vi "provide_OME_data.vi"(6 "image ID":string, 8 "error in (no error)":errorcluster, 9 "structuredAttribute string in":string, 10 "OME element in":refnum<class "XMLElement.lvclass">, 11 "InstrumentDL090324 in":refnum<class "InstrumentDL090324.lvclass">) -> (0 "error out":errorcluster, 1 "structuredAttribute string out":string, 2 "OME element out":refnum<class "XMLElement.lvclass">, 3 "InstrumentDL090324 out":refnum<class "InstrumentDL090324.lvclass">)   [LabVIEW 2010, in "InstrumentDL090324.lvclass"]
uses:
  InstrumentDL090324.lvclass
  common/classes/XMLElement/XMLElement/XMLElement.lvclass
  GenericInstrument/GenericInstrument/GenericInstrument.lvclass
  InstrumentDL090324.lvclass/InstrumentDL090324.ctl
  Detector/GenericDetector/GenericDetector/GenericDetector.lvclass
  LightSource/GenericLightSource/GenericLightSource/GenericLightSource.lvclass
  Objective/GenericObjective/GenericObjective/GenericObjective.lvclass
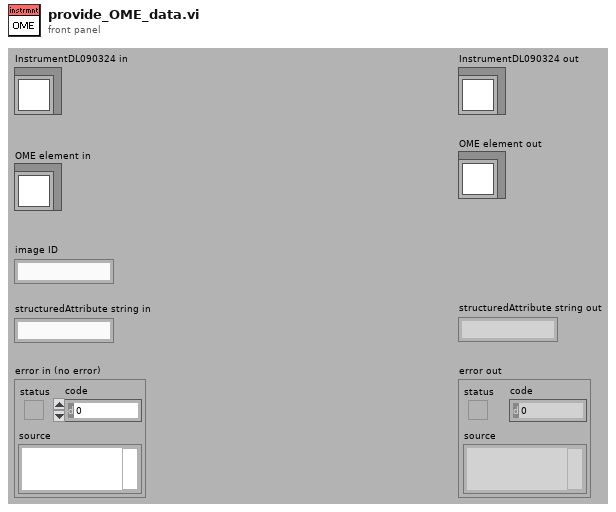
[diagram p1: front panel]
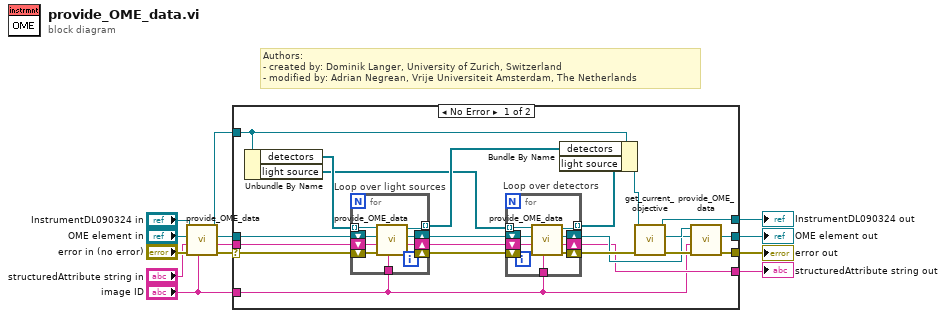
[diagram p0: block diagram]
diagram:
  # "Authors: \n- created by: Dominik Langer, University of Zurich, Switzerland\n- modified by: Adrian Negrean, Vrije Universiteit Amsterdam, The Netherlands"
  n1 = call-parent "provide_OME_data.vi"("image ID"="image ID", "error in (no error)"="error in (no error)", "structuredAttribute string in"="structuredAttribute string in", "OME element in"="OME element in", "GenericPlugin in"="InstrumentDL090324 in") -> ("error out"=w11:errorcluster, "structuredAttribute string out"=w2:string, "OME element out"=w7:refnum<class "XMLElement.lvclass">, "GenericPlugin out"=w8:refnum<class "InstrumentDL090324.lvclass">)  [unwired: 3 in]
  n2 = case shown="No Error" w11 {
    selector: w11 -> [w17 w56]
    tunnel: w8 -> [w14 w55]
    tunnel: w7 -> [w15 w54]
    tunnel: [w30 w56] -> w10
    tunnel: [w29 w54] -> w5
    tunnel: [w18 w55] -> w9
    tunnel: "image ID" -> [w20 _]
    tunnel: w2 -> [w16 w53]
    tunnel: [w21 w53] -> w1
    frame No Error {
      n3 = Unbundle By Name(w14) -> ("detectors"=w34:refnum<class "GenericDetector.lvclass">[], "light source"=w28:refnum<class "GenericLightSource.lvclass">[])
      n4 = for "Loop over light sources" {
        tunnel: w34 -> [w51] mode=indexing
        shift-right: [w48] -> w23
        shift-left: w15 -> [w50]
        shift-right: [w49] -> w25
        shift-left: w17 -> [w52]
        tunnel: [w47] -> w33 mode=indexing
        tunnel: w20 -> [w46]
        shift-right: [w44] -> w24
        shift-left: w16 -> [w45]
        n5 = call-dynamic "provide_OME_data.vi"("image ID"=w46, "error in (no error)"=w52, "structuredAttribute string in"=w45, "OME element in"=w50, "GenericPlugin in"=w51) -> ("error out"=w49:errorcluster, "structuredAttribute string out"=w44:string, "OME element out"=w48:refnum<class "XMLElement.lvclass">, "GenericPlugin out"=w47:refnum<class "GenericDetector.lvclass">)  [unwired: 3 in]
      }
      n6 = for "Loop over detectors" {
        tunnel: w28 -> [w42] mode=indexing
        shift-right: [w39] -> w22
        shift-left: w23 -> [w41]
        shift-right: [w40] -> w26
        shift-left: w25 -> [w43]
        tunnel: [w38] -> w27 mode=indexing
        shift-right: [w36] -> w21
        shift-left: w24 -> [w37]
        tunnel: w20 -> [w35]
        n7 = call-dynamic "provide_OME_data.vi"("image ID"=w35, "error in (no error)"=w43, "structuredAttribute string in"=w37, "OME element in"=w41, "GenericPlugin in"=w42) -> ("error out"=w40:errorcluster, "structuredAttribute string out"=w36:string, "OME element out"=w39:refnum<class "XMLElement.lvclass">, "GenericPlugin out"=w38:refnum<class "GenericLightSource.lvclass">)  [unwired: 3 in]
      }
      n8 = Bundle By Name(cluster=w14, "detectors"=w33, "light source"=w27) -> (w19:refnum<class "InstrumentDL090324.lvclass">)
      n9 = call-dynamic "get_current_objective.vi"("error in (no error)"=w26, "GenericPlugin in"=w19) -> ("error out"=w32:errorcluster, "current objective"=w31:refnum<class "GenericObjective.lvclass">, "GenericPlugin out"=w18:refnum<class "InstrumentDL090324.lvclass">)  [unwired: 7 in]
      n10 = call-dynamic "provide_OME_data.vi"("error in (no error)"=w32, "structuredAttribute string in"=w20, "OME element in"=w22, "GenericObjective in"=w31) -> ("error out"=w30:errorcluster, "OME element out"=w29:refnum<class "XMLElement.lvclass">)  [unwired: 4 in, 2 out]
    }
    frame Error {
    }
  }
  "error out" <- w10
  "InstrumentDL090324 out" <- w9
  "OME element out" <- w5
  "structuredAttribute string out" <- w1
